vi "Load.vi"(8 "error in (no error)":errorcluster, 10 "Data_IN":variant, 11 "ConfigClass_IN":refnum<class "ConfigClass.lvclass">) -> (0 "error out":errorcluster, 3 "ConfigClass_OUT":refnum<class "ConfigClass.lvclass">)   [LabVIEW 2019, in "ConfigClass.lvlib" / "ConfigClass.lvclass"]
uses:
  ConfigClass.lvclass
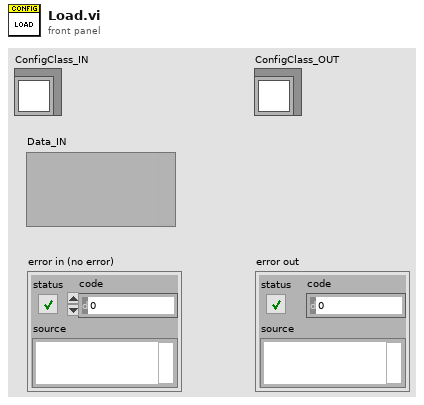
[diagram p1: front panel]
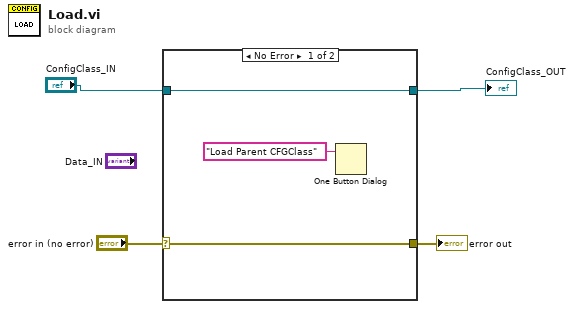
[diagram p0: block diagram]
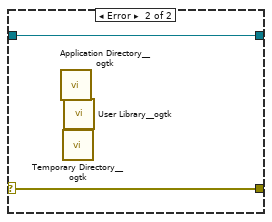
[diagram p2: hidden frame]
diagram:
  n1 = case shown="No Error" "error in (no error)" {
    selector: "error in (no error)" -> [w7 w8]
    tunnel: [w7 w8] -> w3
    tunnel: [w6 w9] -> w1
    tunnel: "ConfigClass_IN" -> [w6 w9]
    frame No Error {
      n2 = One Button Dialog(message="Load Parent CFGClass") -> ()  [unwired: 1 in, 1 out]
    }
    frame Error {
      n3 = call <userlib>:"Application Directory__ogtk.vi"() -> ()  [unwired: 1 in, 1 out]
      n4 = call <userlib>:"Temporary Directory__ogtk.vi"() -> ()  [unwired: 1 in, 1 out]
      n5 = call <userlib>:"User Library__ogtk.vi"() -> ()  [unwired: 1 in, 1 out]
    }
  }
  "error out" <- w3
  "ConfigClass_OUT" <- w1
